vi "Master Sensor Update.vi"(10 "Sensor Reference Input":T3={"LeftMotorEncoderRef"={"DevStatus"={"status"=FALSE, "code"=0, "source"=""}, "EncoderIndex"=enum."Invalid", "CounterIndex"=enum."Invalid", "DistancePerCount"=1.0, "Decoding Type"=enum."4x"}, "RightMotorEncoderRef"={"DevStatus"={"status"=FALSE, "code"=0, "source"=""}, "EncoderIndex"=enum."Invalid", "CounterIndex"=enum."Invalid", "DistancePerCount"=1.0, "Decoding Type"=enum."4x"}, "I2C Gyro"={"DevStatus"={"status"=FALSE, "code"=0, "source"=""}, "Device Address"=0, "Handle"=0, "I2C Bus"=enum."I2C On-Board"}, "Left Shooter Wheel Encoder"={"DevStatus"={"status"=FALSE, "code"=0, "source"=""}, "EncoderIndex"=enum."Enc 0", "CounterIndex"=enum."Ctr 0", "DistancePerCount"=0.0, "Decoding Type"=enum."1x"}, "Ultrasonic AIDeviceRef"={"DevStatus"={"status"=FALSE, "code"=0, "source"=""}, "Analog Channel"=enum."AI 0"}} {"I2C Gyro"."Device Address" format="%.0x"}, 11 "Lights":T1) -> (3 "Sensor Reference Output":T3={"LeftMotorEncoderRef"={"DevStatus"={"status"=FALSE, "code"=0, "source"=""}, "EncoderIndex"=enum."Invalid", "CounterIndex"=enum."Invalid", "DistancePerCount"=1.0, "Decoding Type"=enum."4x"}, "RightMotorEncoderRef"={"DevStatus"={"status"=FALSE, "code"=0, "source"=""}, "EncoderIndex"=enum."Invalid", "CounterIndex"=enum."Invalid", "DistancePerCount"=1.0, "Decoding Type"=enum."4x"}, "I2C Gyro"={"DevStatus"={"status"=FALSE, "code"=0, "source"=""}, "Device Address"=0, "Handle"=0, "I2C Bus"=enum."I2C On-Board"}, "Left Shooter Wheel Encoder"={"DevStatus"={"status"=FALSE, "code"=0, "source"=""}, "EncoderIndex"=enum."Enc 0", "CounterIndex"=enum."Ctr 0", "DistancePerCount"=0.0, "Decoding Type"=enum."1x"}, "Ultrasonic AIDeviceRef"={"DevStatus"={"status"=FALSE, "code"=0, "source"=""}, "Analog Channel"=enum."AI 0"}} {"I2C Gyro"."Device Address" format="%.0x"})   [LabVIEW 2016]
uses:
  Sensor Reference.ctl
  <vilib>/Rock Robotics/WPI/Encoder/WPI_EncoderDevRef.ctl
  <vilib>/Rock Robotics/SystemInterfaces/Encoder/FPGA_EncoderIdx.ctl
  <vilib>/Rock Robotics/SystemInterfaces/Counter/FPGA_CounterCtrSystemIndex.ctl
  <vilib>/Rock Robotics/WPI/Encoder/WPI_EncoderType.ctl
  <vilib>/Rock Robotics/WPI/I2C/WPI_I2CDevRef.ctl
  <vilib>/Rock Robotics/SystemInterfaces/i2clib/i2c_bus.ctl
  <vilib>/Rock Robotics/WPI/AnalogChannel/WPI_AnalogChannelDevRef.ctl
  <vilib>/Rock Robotics/SystemInterfaces/AI/FPGA_AIChannel.ctl
  Light Reference.ctl
  <vilib>/Rock Robotics/WPI/SerialPort/WPI_SerialPortRef.ctl
  Robot Values.vi
  <vilib>/ptbypt/NI_PtbyPt.lvlib
panel:
  out "s? t:f":dbl
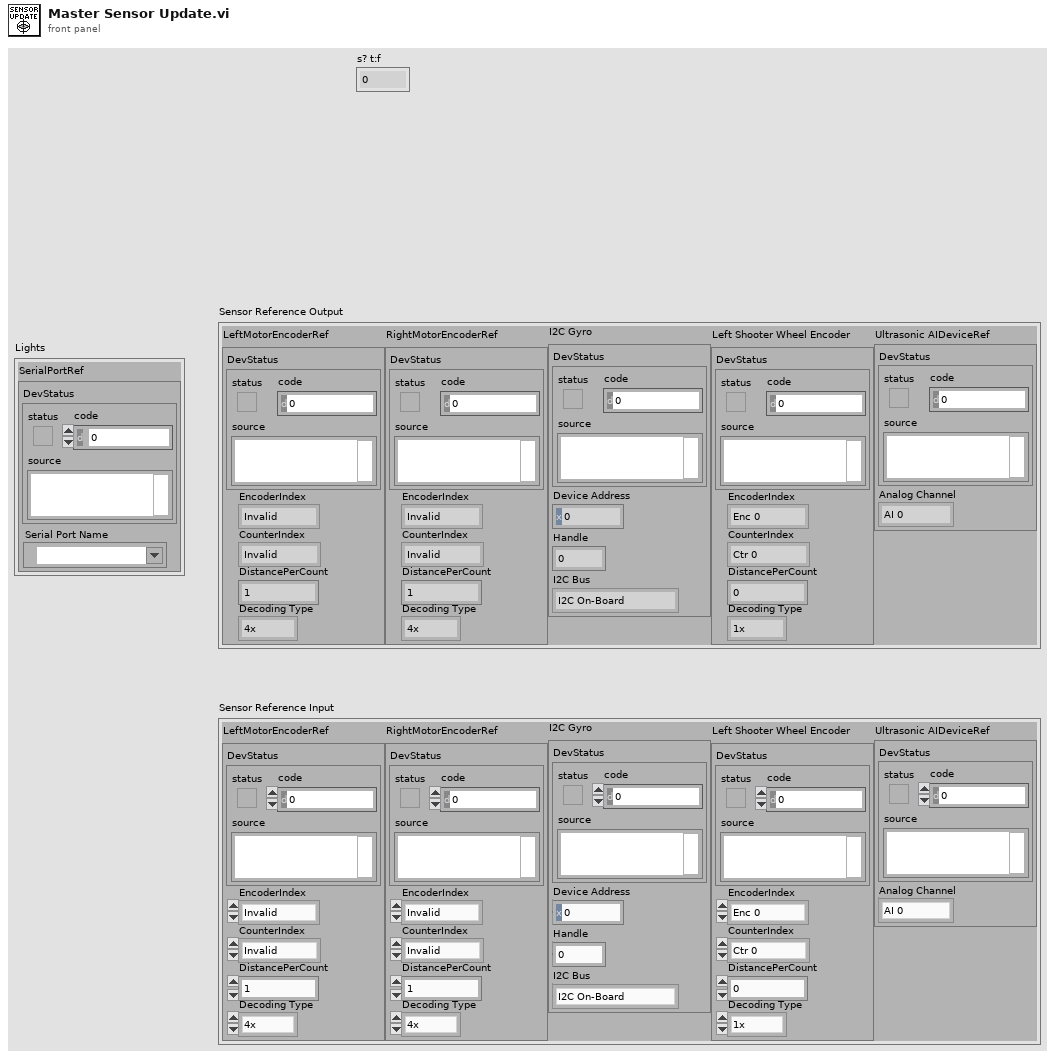
[diagram p1: front panel]
types:
  T1 = typedef "Light Reference.ctl" = cluster{"SerialPortRef":T2}
  T2 = typedef "WPI_SerialPortRef.ctl" = cluster{"DevStatus":errorcluster, "Serial Port Name":refnum<visa-resource-name>}
  T3 = typedef "Sensor Reference.ctl" = cluster{"LeftMotorEncoderRef":T4, "RightMotorEncoderRef":T4, "I2C Gyro":T8, "Left Shooter Wheel Encoder":T4, "Ultrasonic AIDeviceRef":T10}
  T4 = typedef "WPI_EncoderDevRef.ctl" = cluster{"DevStatus":errorcluster, "EncoderIndex":T5, "CounterIndex":T6, "DistancePerCount":dbl, "Decoding Type":T7}
  T5 = typedef "FPGA_EncoderIdx.ctl" = enum8{"Enc 0", "Enc 1", "Enc 2", "Enc 3", "Enc 4", "Enc 5", "Enc 6", "Enc 7", "Invalid"}
  T6 = typedef "FPGA_CounterCtrSystemIndex.ctl" = enum8{"Ctr 0", "Ctr 1", "Ctr 2", "Ctr 3", "Ctr 4", "Ctr 5", "Ctr 6", "Ctr 7", "Invalid"}
  T7 = typedef "WPI_EncoderType.ctl" = enum16{"1x", "2x", "4x"}
  T8 = typedef "WPI_I2CDevRef.ctl" = cluster{"DevStatus":errorcluster, "Device Address":u8, "Handle":i32, "I2C Bus":T9}
  T9 = typedef "i2c_bus.ctl" = enum16{"I2C On-Board", "I2C MXP", "Invalid"}
  T10 = typedef "WPI_AnalogChannelDevRef.ctl" = cluster{"DevStatus":errorcluster, "Analog Channel":T11}
  T11 = typedef "FPGA_AIChannel.ctl" = enum8{"AI 0", "AI 1", "AI 2", "AI 3", "AI MXP 0", "AI MXP 1", "AI MXP 2", "AI MXP 3", "Invalid"}
  T12 = typedef "Robot Values.ctl" = cluster{"Robot Drive":cluster{"Left Motor Power":dbl, "Right Motor Power":dbl, "Left Encoder Value":dbl, "Right Encoder Value":dbl, "High Gear?":bool, "PTO?":bool}, "Sensors":cluster{"Gyro Angle":u16, "Recalibrate Gyro":bool, "Reset Gyro":bool, "Ultrasonic":dbl}, "Shooter":cluster{"Prep Wheels":bool, "Shoot":bool, "Left Shooter Wheel Speed":dbl, "Wheels Moving":bool, "Shooter Prepped":bool, "Shooter RPS SP":dbl, "Shooting?":bool, "Left Shooter Wheel Power":dbl, "Right Shooter Wheel Power":dbl, "Acquisition Conveyor Power":dbl, "Hopper Beater Bar Power":dbl, "Filtered Left Shooter Speed":dbl, "Acquisition Motor Power":dbl, "Joystick Add":dbl, "D-Pad Add":dbl, "Shooter Use PID?":bool}, "Robot States":cluster{"Drive mode":string, "Alliance":T13, "Position":T14}, "Gear":cluster{"Ejection Active":bool}}
  T13 = typedef "WPI_DriverStationAllianceInfo.ctl" = enum16{"Red", "Blue", "Invalid"}
  T14 = typedef "WPI_DriverStationPositionInfo.ctl" = enum16{"1", "2", "3"}
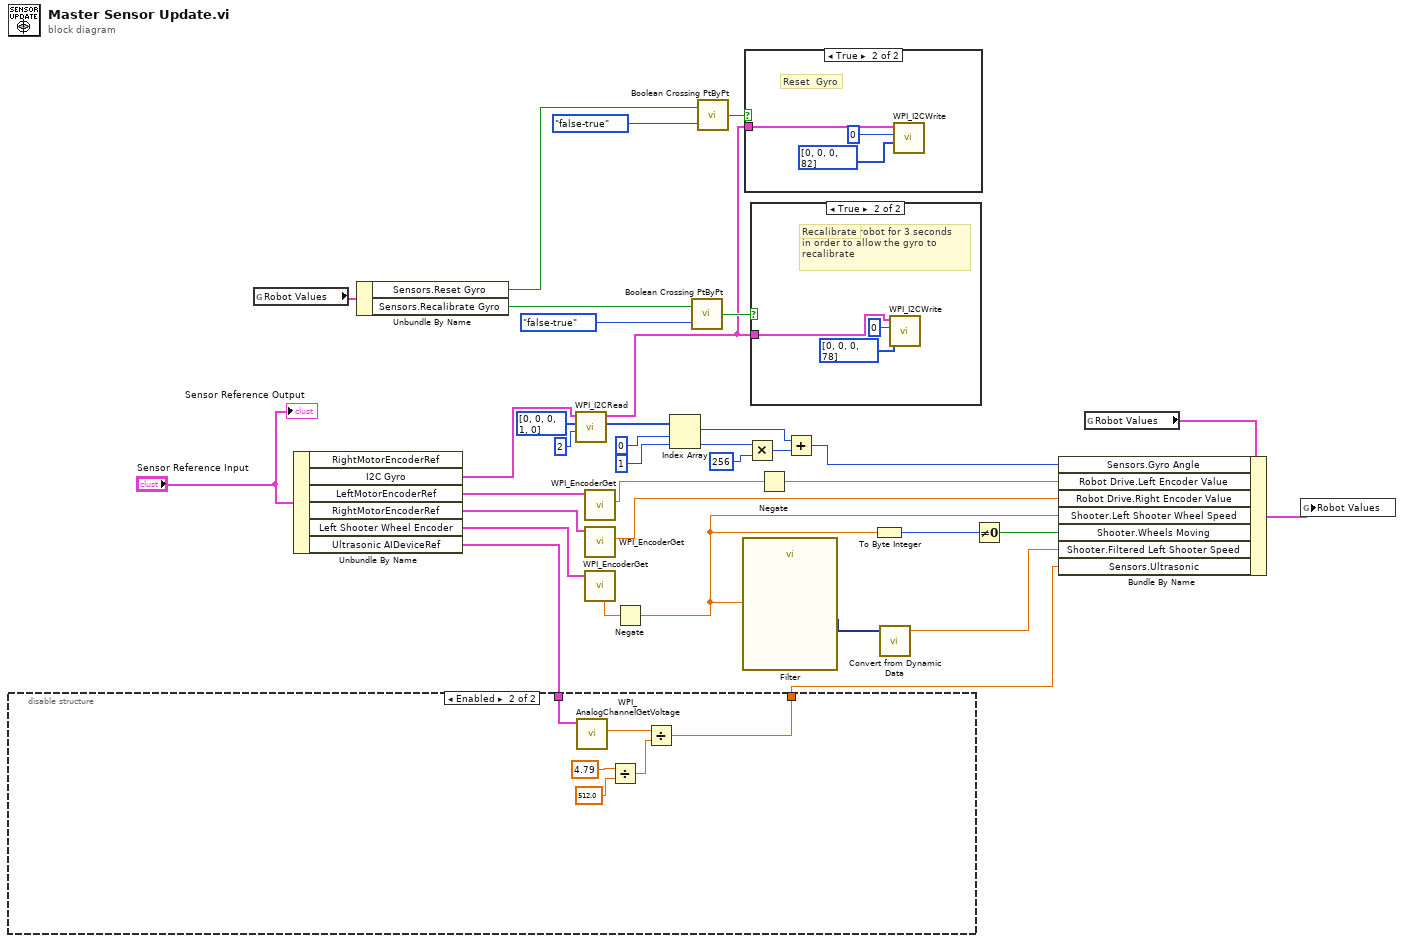
[diagram p0: block diagram]
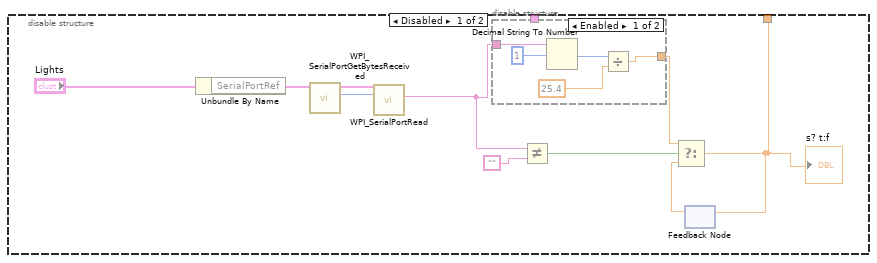
[diagram p2: hidden frame]
diagram:
  n1 = global read "Robot Values.vi" "Robot Values"() -> (w20:T12)
  n2 = Unbundle By Name("Sensor Reference Input") -> ("I2C Gyro"=w19:T8, "LeftMotorEncoderRef"=w33:T4, "RightMotorEncoderRef"=w31:T4, "Left Shooter Wheel Encoder"=w9:T4, "Ultrasonic AIDeviceRef"=w2:T10)  [unwired: 1 out]
  n3 = disable-structure shown="Enabled" {
    disable-tunnel: [w37 w56] -> w3
    disable-tunnel: w2 -> [_ w58]
    frame Disabled {
      n4 = Unbundle By Name("Lights") -> ("SerialPortRef"=w44:T2)
      n5 = call <vilib>:"WPI_SerialPortGetBytesReceived.vi"("SerialPortRef"=w44) -> ("Bytes at Port"=w46:u32, "SerialPortRef"=w45:T2)  [unwired: 8 in, 1 out]
      n6 = call <vilib>:"WPI_SerialPortRead.vi"("Num Bytes to Read"=w46, "SerialPortRef"=w45) -> ("Buffer"=w39:string)  [unwired: 7 in, 2 out]
      n7 = disable-structure shown="Enabled" {
        disable-tunnel: w39 -> [w51 w52]
        disable-tunnel: [w48 w52] -> w38
        frame Enabled {
          n8 = Decimal String To Number(string=w51, offset=1 ("offset (0)")) -> (number=w49:i32)  [unwired: 1 in, 1 out]
          n9 = Divide(x=w49, y=25.4) -> (x/y=w48:dbl)
        }
        frame Disabled {
        }
      }
      n10 = Not Equal?(x=w39, y="") -> (x != y?=w41:bool)
      n11 = feedback #1() -> (w40:dbl)  [unwired: 1 in]
      n12 = Select(t=w38, s=w41, f=w40) -> (s? t:f=w37:dbl)
      "s? t:f" <- w37
      n13 = feedback-in #1(w37) -> ()
    }
    frame Enabled {
      n14 = call <vilib>:"WPI_AnalogChannelGetVoltage.vi"("AIDeviceRef"=w58) -> ("Voltage"=w57:dbl)  [unwired: 8 in, 2 out]
      n15 = Divide(x=4.79, y=512.0) -> (x/y=w55:dbl)
      n16 = Divide(x=w57, y=w55) -> (x/y=w56:dbl)
    }
  }
  n17 = Unbundle By Name(w20) -> ("Sensors.Reset Gyro"=w13:bool, "Sensors.Recalibrate Gyro"=w18:bool)
  n18 = call <vilib>:"WPI_I2CRead.vi"("I2CBytesToRead"=u8 2, "I2CRegister"=u8[] [0, 0, 0, 1, 0], "I2CDevRef"=w19) -> ("Data Out"=w28:u8[], "I2CDevRef"=w11:T8)  [unwired: 6 in, 1 out]
  n19 = call <vilib>:"WPI_EncoderGet.vi"("EncoderDevRef"=w33) -> ("Distance"=w32:dbl)  [unwired: 5 in, 5 out]
  n20 = call <vilib>:"WPI_EncoderGet.vi"("EncoderDevRef"=w31) -> ("Distance"=w10:dbl)  [unwired: 5 in, 5 out]
  n21 = call <vilib>:"WPI_EncoderGet.vi"("EncoderDevRef"=w9) -> ("Rate"=w4:dbl)  [unwired: 5 in, 5 out]
  n22 = Negate(x=w4) -> (-x=w1:dbl)
  n23 = Index Array(array=w28, index #1=0 ("index"), index #2=1 ("index")) -> (element #1=w23:u8, element #2=w25:u8)
  n24 = call <vilib>:"Boolean Crossing PtByPt.vi"("direction"=enum16{"either", "false-true", "true-false"}."false-true", "input"=w18) -> ("crossing"=w17:bool)  [unwired: 1 in]
  n25 = call <vilib>:"Boolean Crossing PtByPt.vi"("direction"=enum16{"either", "false-true", "true-false"}."false-true", "input"=w13) -> ("crossing"=w14:bool)  [unwired: 1 in]
  n26 = call "Filter"("Signal"=w1) -> ("Filtered Signal"=w6:dynamicdata)  [unwired: 9 in, 1 out]
  n27 = case shown="True" w14 {
    tunnel: w11 -> [_ w59]
    frame False {
    }
    frame True {
      # "Reset  Gyro"
      n28 = call <vilib>:"WPI_I2CWrite.vi"("I2CDataToSend"=u8[] [0, 0, 0, 82], "I2CRegister"=u8 0, "I2CDevRef"=w59) -> ()  [unwired: 7 in, 2 out]
    }
  }
  n29 = Multiply(x=w25, y=u16 256) -> (x*y=w22:u16)
  n30 = case shown="True" w17 {
    tunnel: w11 -> [_ w62]
    frame False {
    }
    frame True {
      # "Recalibrate"
      # "Don't move robot for 3 seconds\nin order to allow the gyro to\nrecalibrate"
      n31 = call <vilib>:"WPI_I2CWrite.vi"("I2CDataToSend"=u8[] [0, 0, 0, 78], "I2CRegister"=u8 0, "I2CDevRef"=w62) -> ()  [unwired: 7 in, 2 out]
    }
  }
  n32 = Negate(x=w32) -> (-x=w15:dbl)
  n33 = Add(x=w23, y=w22) -> (x+y=w21:u16)
  n34 = To Byte Integer(number=w1) -> (8bit integer=w7:i8)
  n35 = call "Convert from Dynamic Data"("Dynamic Data Type"=w6) -> ("Scalar"=w5:dbl)  [unwired: 3 in]
  n36 = Not Equal To 0?(x=w7) -> (x != 0?=w8:bool)
  n37 = global read "Robot Values.vi" "Robot Values"() -> (w35:T12)
  n38 = Bundle By Name(cluster=w35, "Sensors.Gyro Angle"=w21, "Robot Drive.Left Encoder Value"=w15, "Robot Drive.Right Encoder Value"=w10, "Shooter.Left Shooter Wheel Speed"=w1, "Shooter.Wheels Moving"=w8, "Shooter.Filtered Left Shooter Speed"=w5, "Sensors.Ultrasonic"=w3) -> (w36:T12)
  n39 = global write "Robot Values.vi" "Robot Values"(w36) -> ()
  "Sensor Reference Output" <- "Sensor Reference Input"
